vi "String_to_XYZ_Pos.vi"(2 "Input string":string, 4 "Position label":string) -> (1 "Some labels found":bool, 5 "X":dbl format="%.2f", 6 "Y":dbl format="%.2f", 7 "Z":dbl format="%.2f")   [LabVIEW 2011]
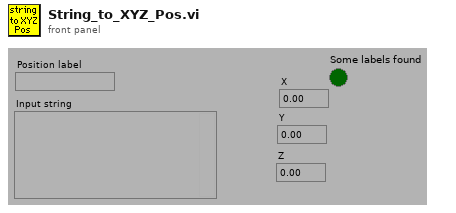
[diagram p1: front panel]
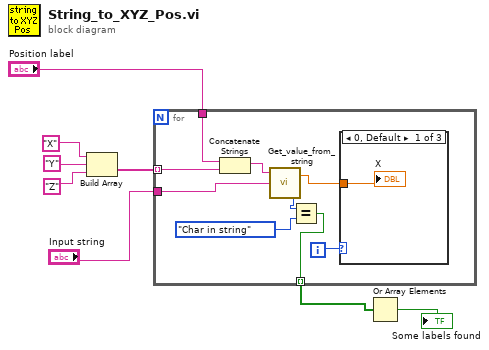
[diagram p0: block diagram]
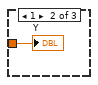
[diagram p2: hidden frame]
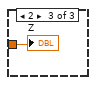
[diagram p3: hidden frame]
diagram:
  n1 = Build Array("X", "Y", "Z") -> (w8:string[])
  n2 = for {
    tunnel: "Position label" -> [w12]
    tunnel: w8 -> [w17] mode=indexing
    tunnel: "Input string" -> [w15]
    tunnel: [w9] -> w2 mode=indexing
    i -> [w14]
    n3 = Concatenate Strings(w12, w17) -> (w16:string)
    n4 = call "Get_value_from_string.vi"("Input string"=w15, "Variable name"=w16) -> ("Status"=w11:enum16{"Char in string", "Char not in string"}, "Value"=w13:dbl)  [unwired: 1 in]
    n5 = Equal?(x=w11, y=enum16{"Char in string", "Char not in string"}."Char in string" ("Status")) -> (x = y?=w9:bool)
    n6 = case shown="0, Default" w14 {
      tunnel: w13 -> [w18 w19 w20]
      frame 0, Default {
        "X" <- w18
      }
      frame 1 {
        "Y" <- w19
      }
      frame 2 {
        "Z" <- w20
      }
    }
  }
  n7 = Or Array Elements(Boolean array=w2) -> (logical OR=→"Some labels found":bool)
